vi "PH_Beckhoff_PP_PU.calc RR State.vi"(1 "old RR Status":T1 items=["no info", "off/false/out", "on/true/in", "Failure", "Alarm", "Status 1", "Status 2", "Status 3"], 2 "GUI Refs: open and closed":refnum<vi>[](array[refnum]), 3 "# in Data: open and closed":i32[](array[numeric]), 4 "Digital Inputs":T2, 5 "error in":errorcluster) -> (17 "Ross Relais Status":T1 items=["no info", "off/false/out", "on/true/in", "Failure", "Alarm", "Status 1", "Status 2", "Status 3"], 19 "error out":errorcluster)   [LabVIEW 2014, in "PH_Beckhoff_PP_PU.lvlib"]
doc: "This VI calculates the RR status and sets the RR Input GUI element."
uses:
  PH_Beckhoff_PP_PU.lvlib
  PH_StatusHandler/PH_StatusHandler.Status.ctl
  PH_Beckhoff/PH_Beckhoff.Digital Inputs.ctl
  PH_StatusHandler/PH_StatusHandler.lvlib
  PH_Common/PH_Common.lvlib
  PH_Beckhoff/PH_Beckhoff.lvlib
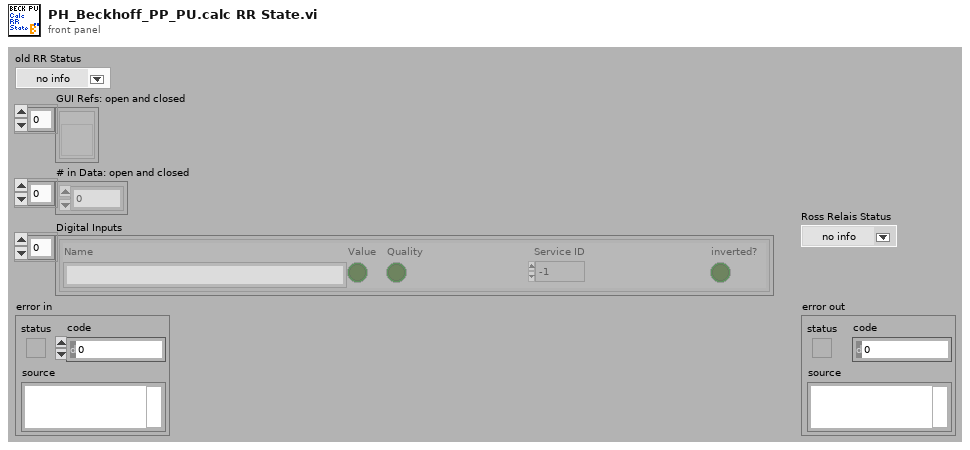
[diagram p1: front panel]
types:
  T1 = typedef "PH_StatusHandler.lvlib/PH_StatusHandler.Status.ctl" = i16
  T2 = typedef "PH_Beckhoff.lvlib/PH_Beckhoff.Digital Inputs.ctl" = cluster{"Name":string, "Value":bool, "Quality":bool, "Service ID":i32, "inverted?":bool}[]
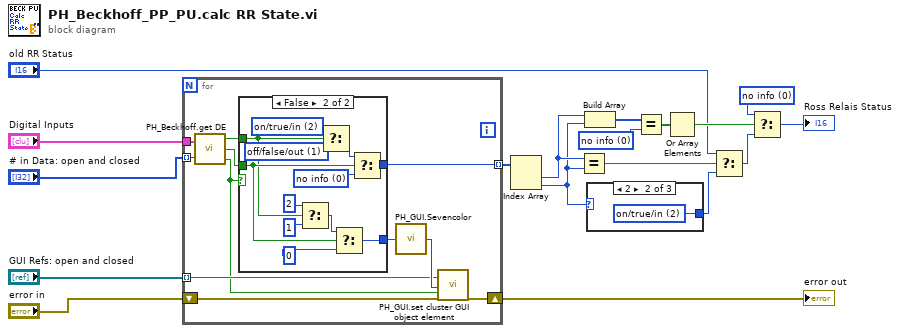
[diagram p0: block diagram]
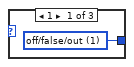
[diagram p2: hidden frame]
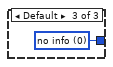
[diagram p3: hidden frame]
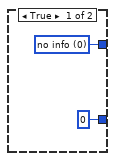
[diagram p4: hidden frame]
diagram:
  w10 = T1 0 items=["no info", "off/false/out", "on/true/in", "Failure", "Alarm", "Status 1", "Status 2", "Status 3"] ("Ignitron Status")
  w17 = T1 0 items=["no info", "off/false/out", "on/true/in", "Failure", "Alarm", "Status 1", "Status 2", "Status 3"] ("State RR open")
  n1 = for {
    tunnel: [w29] -> w18 mode=indexing
    tunnel: "Digital Inputs" -> [w28]
    tunnel: "# in Data: open and closed" -> [w27] mode=indexing
    shift-right: [w23] -> w6
    shift-left: "error in" -> [w22]
    tunnel: "GUI Refs: open and closed" -> [w21] mode=indexing
    n2 = call "PH_Beckhoff.get DE.vi"("Digital Values"=w28, "index of element"=w27) -> ("Value"=w19:bool, "Quality"=w26:bool, "Tag not found"=w20:bool)
    n3 = case shown="False" w20 {
      tunnel: [w31 w43] -> w29
      tunnel: w26 -> [_ w34]
      tunnel: w19 -> [_ w33]
      tunnel: [0 ("State") w32] -> w25
      frame True {
        w31 = T1 0 items=["no info", "off/false/out", "on/true/in", "Failure", "Alarm", "Status 1", "Status 2", "Status 3"] ("HV On State")
      }
      frame False {
        w39 = T1 1 items=["no info", "off/false/out", "on/true/in", "Failure", "Alarm", "Status 1", "Status 2", "Status 3"] ("HV On State")
        w40 = T1 2 items=["no info", "off/false/out", "on/true/in", "Failure", "Alarm", "Status 1", "Status 2", "Status 3"] ("HV On State")
        w42 = T1 0 items=["no info", "off/false/out", "on/true/in", "Failure", "Alarm", "Status 1", "Status 2", "Status 3"] ("HV On State")
        n4 = Select(t=2 ("State"), s=w33, f=1 ("State")) -> (s? t:f=w38:i32)
        n5 = Select(t=w40, s=w33, f=w39) -> (s? t:f=w41:T1)
        n6 = Select(t=w38, s=w34, f=0 ("State")) -> (s? t:f=w32:i32)
        n7 = Select(t=w41, s=w34, f=w42) -> (s? t:f=w43:T1)
      }
    }
    n8 = call "PH_GUI.Sevencolor.vi"("State"=w25) -> ("Color Box"=w24:u32)
    n9 = call "PH_GUI.set cluster GUI object element.vi"("Ctl Refnum"=w21, "Value"=w24, "Blinking? (false)"=w20, "error in"=w22) -> ("error out"=w23:errorcluster)  [unwired: 15 in]
  }
  "error out" <- w6
  n10 = Index Array(array=w18) -> (element #1=w11:T1, element #2=w9:T1)  [unwired: 2 in]
  n11 = Equal?(x=w11, y=w9) -> (x = y?=w14:bool)
  n12 = Build Array(w11, w9) -> (w13:T1[])
  n13 = case shown="2" w9 {
    tunnel: [w44 w45 w46] -> w8
    frame 1 {
      w44 = T1 1 items=["no info", "off/false/out", "on/true/in", "Failure", "Alarm", "Status 1", "Status 2", "Status 3"] ("Ignitron Status")
    }
    frame 2 {
      w45 = T1 2 items=["no info", "off/false/out", "on/true/in", "Failure", "Alarm", "Status 1", "Status 2", "Status 3"] ("Ignitron Status")
    }
    frame Default {
      w46 = T1 0 items=["no info", "off/false/out", "on/true/in", "Failure", "Alarm", "Status 1", "Status 2", "Status 3"] ("Ignitron Status")
    }
  }
  n14 = Equal?(x=w13, y=w17) -> (x = y?=w16:bool[])
  n15 = Or Array Elements(Boolean array=w16) -> (logical OR=w15:bool)
  n16 = Select(t="old RR Status", s=w14, f=w8) -> (s? t:f=w12:T1)
  n17 = Select(t=w10, s=w15, f=w12) -> (s? t:f=→"Ross Relais Status":T1)
